vi "CreateHardwareActionQueues.vi"(8 "Error In":errorcluster) -> (0 "Error Out":errorcluster, 3 "Hardware Action Queues":T1)   [LabVIEW 2012]
uses:
  HeaterAction.ctl
  libs/Application.lvlib
  HeaterActionQueueElement.ctl
  MFCAction.ctl
  MFCActionQueueElement.ctl
  HardwareActionQueues.ctl
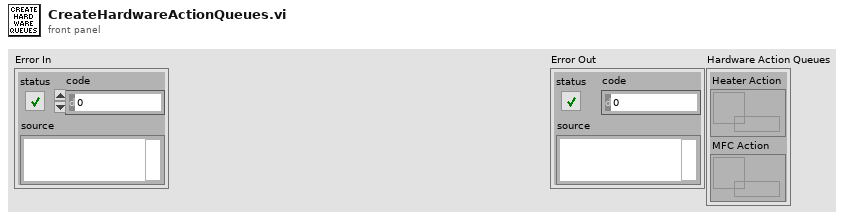
[diagram p1: front panel]
types:
  T1 = typedef "Application.lvlib/HardwareActionQueues.ctl" = cluster{"Heater Action":refnum<queue>, "MFC Action":refnum<queue>}
  T2 = typedef "Application.lvlib/HeaterActionQueueElement.ctl" = cluster{"Action":T3, "Data":variant}
  T3 = typedef "Application.lvlib/HeaterAction.ctl" = enum16{"Initialize", "Start", "Read", "Write", "Stop", "Shutdown"}
  T4 = typedef "Application.lvlib/MFCActionQueueElement.ctl" = cluster{"Action":T5, "Data":variant}
  T5 = typedef "Application.lvlib/MFCAction.ctl" = enum16{"Initialize", "Start", "Read", "Write", "Stop", "Shutdown"}
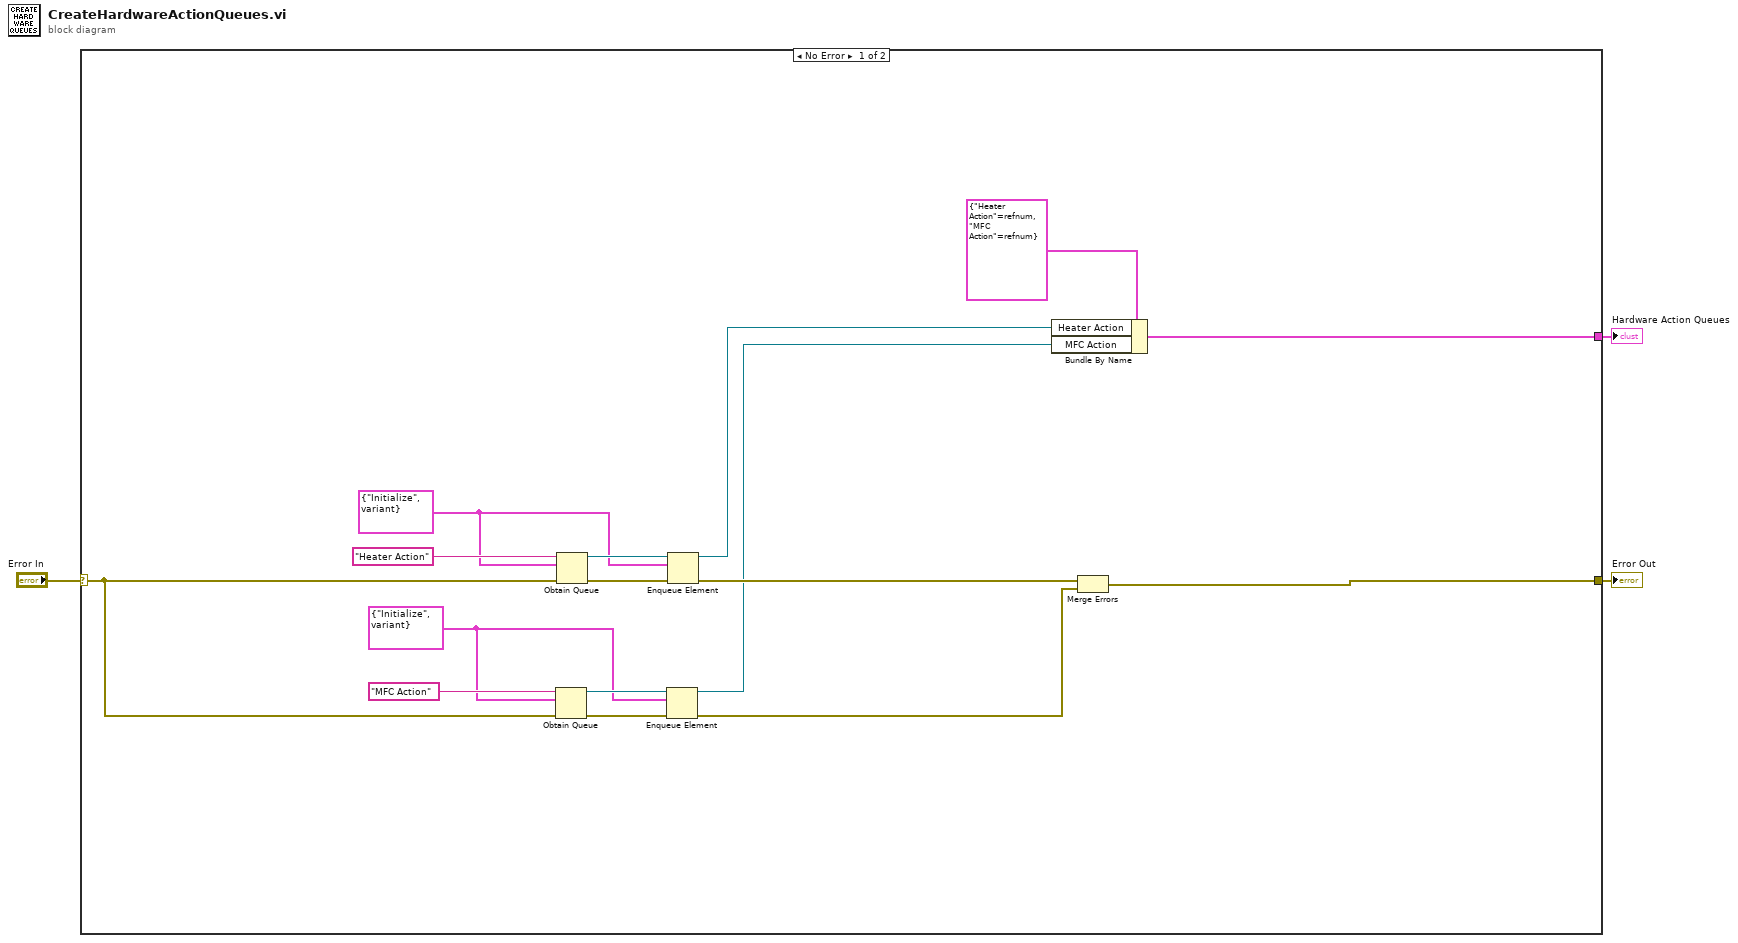
[diagram p0: block diagram]
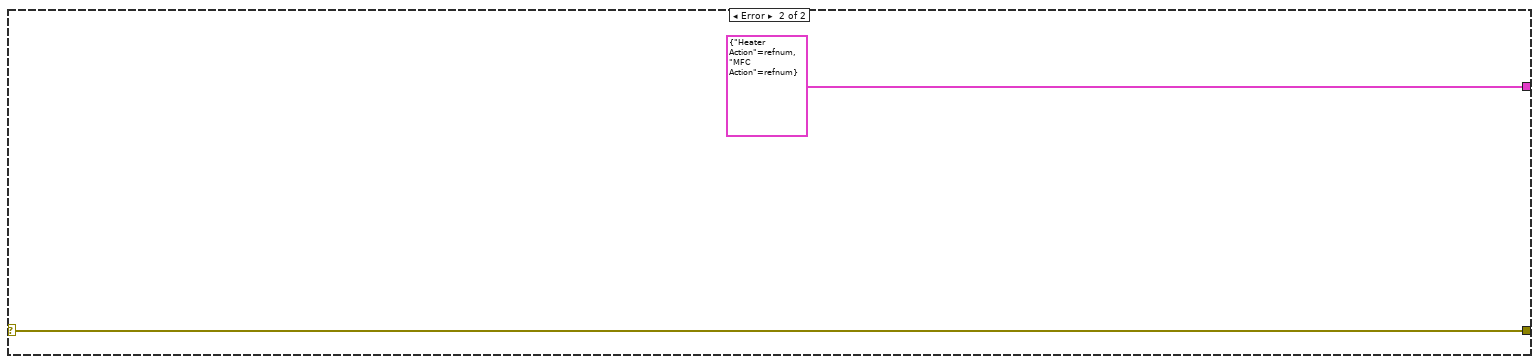
[diagram p2: hidden frame]
diagram:
  n1 = case shown="No Error" "Error In" {
    selector: "Error In" -> [w12 w21]
    tunnel: [w9 w21] -> w2
    tunnel: [w6 T1 {"Heater Action"=refnum, "MFC Action"=refnum} ("Hardware Action Queues")] -> w1
    frame No Error {
      w5 = T2 {"Action"=enum."Initialize", "Data"=variant} ("Heater Action Queue Element")
      w4 = T4 {"Action"=enum."Initialize", "Data"=variant} ("MFC Action Queue Element")
      n2 = Obtain Queue(name (unnamed)="MFC Action", element data type=w4, error in (no error)=w12) -> (queue out=w16:refnum<queue>, error out=w15:errorcluster)  [unwired: 2 in, 1 out]
      n3 = Obtain Queue(name (unnamed)="Heater Action", element data type=w5, error in (no error)=w12) -> (queue out=w18:refnum<queue>, error out=w17:errorcluster)  [unwired: 2 in, 1 out]
      n4 = Enqueue Element(queue=w16, element=w4, error in (no error)=w15) -> (queue out=w7:refnum<queue>, error out=w10:errorcluster)  [unwired: 1 in, 1 out]
      n5 = Enqueue Element(queue=w18, element=w5, error in (no error)=w17) -> (queue out=w8:refnum<queue>, error out=w11:errorcluster)  [unwired: 1 in, 1 out]
      n6 = Bundle By Name(cluster=T1 {"Heater Action"=refnum, "MFC Action"=refnum} ("Hardware Action Queues"), "Heater Action"=w8, "MFC Action"=w7) -> (w6:T1)
      n7 = Merge Errors(w11, w10) -> (w9:errorcluster)
    }
    frame Error {
    }
  }
  "Error Out" <- w2
  "Hardware Action Queues" <- w1
